vi "Pockels Cal-Objective setting reminder.vi"(11 "Message in":string) -> (3 "Message":string)   [LabVIEW 2013]
uses:
  Globals/gl_Calibration globals.vi
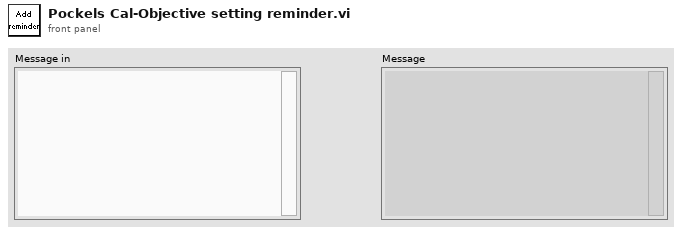
[diagram p1: front panel]
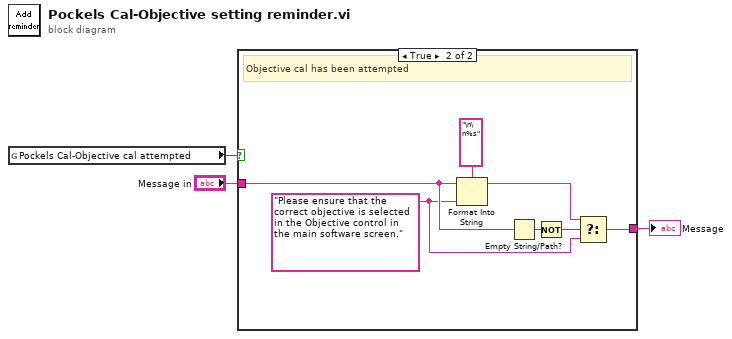
[diagram p0: block diagram]
diagram:
  n1 = global read "gl_Calibration globals.vi" "Pockels Cal-Objective cal attempted"() -> (w2:bool)
  n2 = case shown="True" w2 {
    tunnel: "Message in" -> [w4 w6]
    tunnel: [w4 w7] -> w3
    frame False {
      # "Objective cal has not been attempted"
    }
    frame True {
      w5 = "Please ensure that the correct objective is selected in the Objective control in the main software screen." ("input 1")
      # "Objective cal has been attempted"
      n3 = Format Into String(format string="\n\n%s", initial string=w6, w5) -> (resulting string=w8:string)  [unwired: 1 in, 1 out]
      n4 = Empty String/Path?(string/path=w6) -> (empty?=w10:bool)
      n5 = Not(x=w10) -> (.not. x?=w9:bool)
      n6 = Select(t=w8, s=w9, f=w5) -> (s? t:f=w7:string)
    }
  }
  "Message" <- w3
